vi "Init_Sylap.vi"(0 "VISA resource name":refnum<visa-resource-name>, 1 "LaserMaxCount":u64=10, 2 "LaserHalfLength":u64=9, 3 "TotalOffset":u64, 4 "PulseLength":u64=10, 5 "error in (no error)":errorcluster) -> (8 "maxPulseLength (ps)":i32, 10 "maxPulseLength":i32, 14 "VISA resource name out":refnum<visa-resource-name>, 15 "Decimation":dbl, 16 "simLaser freq. (MHz)":dbl, 17 "TotalOffset (ps)":dbl, 18 "Length Pulse (ps)":dbl, 19 "error out":errorcluster)   [LabVIEW 2020]
uses:
  <vilib>/Instr/_visa.llb/VISA Configure Serial Port (Instr).vi
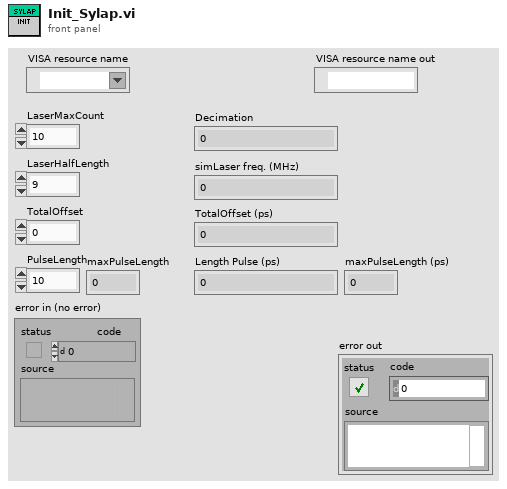
[diagram p1: front panel]
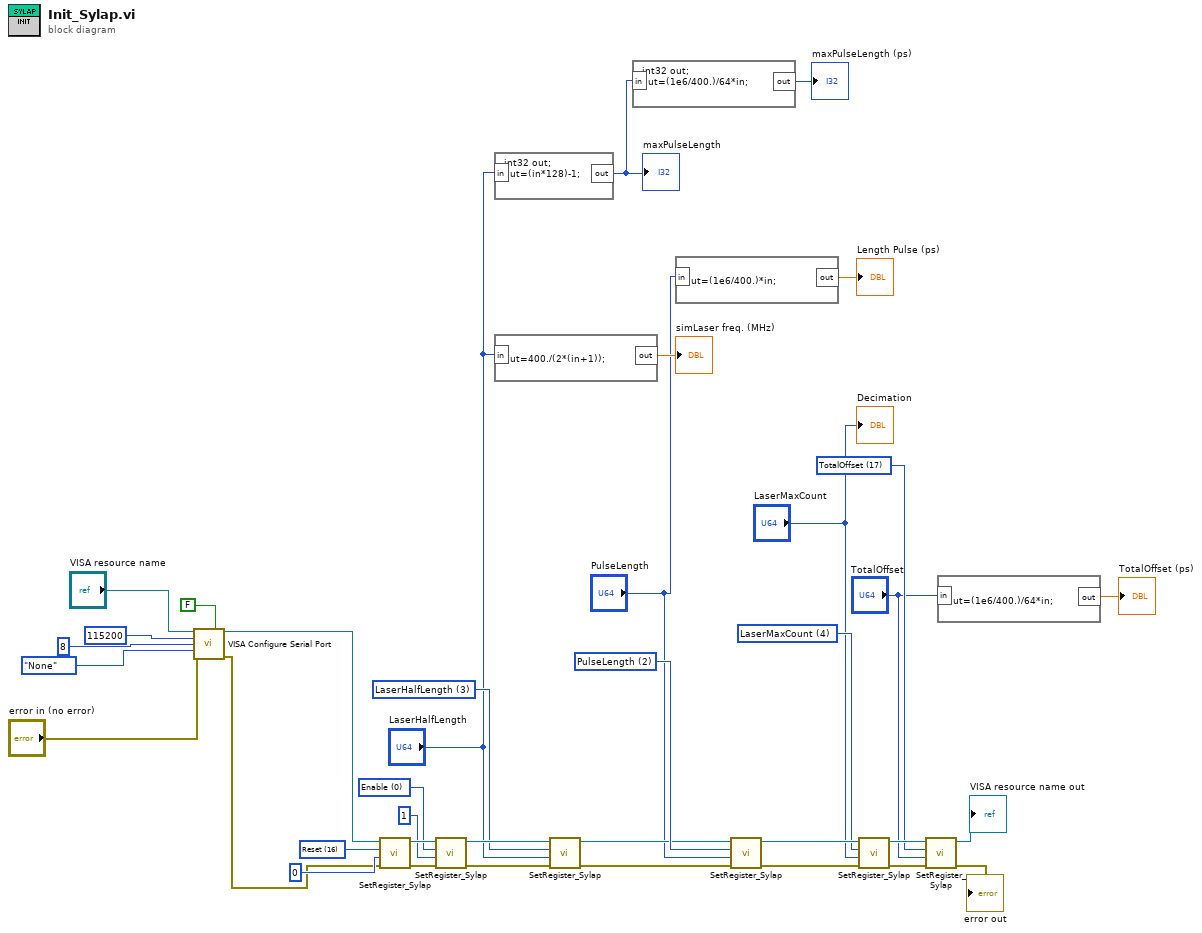
[diagram p0: block diagram]
diagram:
  w21 = u16 17 items=["Enable"=0, "TotalOffsetCoarse"=1, "PulseLength"=2, "LaserHalfLength"=3, "LaserMaxCount"=4, "TotalOffset"=17, "ResetCounters"=18, "Reset"=16] ("Register Name")
  w18 = u16 4 items=["Enable"=0, "TotalOffsetCoarse"=1, "PulseLength"=2, "LaserHalfLength"=3, "LaserMaxCount"=4, "TotalOffset"=17, "ResetCounters"=18, "Reset"=16] ("Register Name")
  w28 = u16 2 items=["Enable"=0, "TotalOffsetCoarse"=1, "PulseLength"=2, "LaserHalfLength"=3, "LaserMaxCount"=4, "TotalOffset"=17, "ResetCounters"=18, "Reset"=16] ("Register Name")
  w29 = u16 3 items=["Enable"=0, "TotalOffsetCoarse"=1, "PulseLength"=2, "LaserHalfLength"=3, "LaserMaxCount"=4, "TotalOffset"=17, "ResetCounters"=18, "Reset"=16] ("Register Name")
  w32 = u16 0 items=["Enable"=0, "TotalOffsetCoarse"=1, "PulseLength"=2, "LaserHalfLength"=3, "LaserMaxCount"=4, "TotalOffset"=17, "ResetCounters"=18, "Reset"=16] ("Register Name")
  w37 = u16 16 items=["TotalOffsetCoarse"=1, "PulseLength"=2, "LaserHalfLength"=3, "LaserMaxCount"=4, "TotalOffset"=17, "ResetCounters"=0, "Reset"=16] ("Register Name")
  n1 = call-poly "VISA Configure Serial Port"("VISA resource name"="VISA resource name", "Enable Termination\nChar (T)"=FALSE ("Enable Termination\nChar (T)"), "baud rate (9600)"=u32 115200, "data bits (8)"=u16 8, "parity (0:none)"=enum16{"None", "Odd", "Even", "Mark", "Space"}."None", "error in (no error)"="error in (no error)") -> ("VISA resource name out"=w13:refnum<visa-resource-name>, "error out"=w12:errorcluster)  [unwired: 8 in]
  n2 = call "SetRegister_Sylap.vi"("error in (no error)"=w12, "Input Value"=u64 0, "Register Name"=w37, "VISA resource name"=w13) -> ("error out"=w35:errorcluster, "VISA resource name out"=w34:refnum<visa-resource-name>)  [unwired: 4 in, 2 out]
  n3 = call "SetRegister_Sylap.vi"("error in (no error)"=w35, "Input Value"=u64 1, "Register Name"=w32, "VISA resource name"=w34) -> ("error out"=w31:errorcluster, "VISA resource name out"=w30:refnum<visa-resource-name>)  [unwired: 4 in, 2 out]
  n4 = formula code="int32 out;\nout=(in*128)-1;"("in"="LaserHalfLength") -> ("out"=w2:i32)
  "maxPulseLength" <- w2
  n5 = formula code="out=400./(2*(in+1));"("in"="LaserHalfLength") -> ("out"=→"simLaser freq. (MHz)":dbl)
  n6 = call "SetRegister_Sylap.vi"("error in (no error)"=w31, "Input Value"="LaserHalfLength", "Register Name"=w29, "VISA resource name"=w30) -> ("error out"=w26:errorcluster, "VISA resource name out"=w27:refnum<visa-resource-name>)  [unwired: 4 in, 2 out]
  n7 = formula code="int32 out;\nout=(1e6/400.)/64*in;"("in"=w2) -> ("out"=→"maxPulseLength (ps)":i32)
  n8 = formula code="out=(1e6/400.)*in;"("in"="PulseLength") -> ("out"=→"Length Pulse (ps)":dbl)
  n9 = call "SetRegister_Sylap.vi"("error in (no error)"=w26, "Input Value"="PulseLength", "Register Name"=w28, "VISA resource name"=w27) -> ("error out"=w25:errorcluster, "VISA resource name out"=w24:refnum<visa-resource-name>)  [unwired: 4 in, 2 out]
  n10 = call "SetRegister_Sylap.vi"("error in (no error)"=w25, "Input Value"="LaserMaxCount", "Register Name"=w18, "VISA resource name"=w24) -> ("error out"=w23:errorcluster, "VISA resource name out"=w22:refnum<visa-resource-name>)  [unwired: 4 in, 2 out]
  n11 = call "SetRegister_Sylap.vi"("error in (no error)"=w23, "Input Value"="TotalOffset", "Register Name"=w21, "VISA resource name"=w22) -> ("error out"=→"error out":errorcluster, "VISA resource name out"=→"VISA resource name out":refnum<visa-resource-name>)  [unwired: 4 in, 2 out]
  n12 = formula code="out=(1e6/400.)/64*in;"("in"="TotalOffset") -> ("out"=→"TotalOffset (ps)":dbl)
  "Decimation" <- "LaserMaxCount"
